vi "Test Video.vi"() -> ()   [LabVIEW 2015]
uses:
  Controls/Video Resolution Control.ctl
  Controls/Led Control.ctl
  Controls/Video Format Control.ctl
  <vilib>/Analysis/baseanly.llb/Mean (DBL).vi
  <vilib>/myRIO/Common/Instrument Driver Framework/myRIO v1.0/UART/vis/myRIO v1.0 Close UART.vi
  <vilib>/myRIO/Common/Instrument Driver Framework/Utilities/vis/FPGA Ref Manager.vi
  <vilib>/myRIO/Common/Instrument Driver Framework/myRIO v1.0/myRIO v1.0 Reset FPGA.vi
  <vilib>/myRIO/Common/Instrument Driver Framework/myRIO v1.0/IRQ/vis/myRIO v1.0 IRQ Info FGV.vi
  <vilib>/myRIO/Common/Instrument Driver Framework/myRIO v1.0/IRQ/vis/myRIO v1.0 Timer IRQ Info FGV.vi
  <vilib>/myRIO/Common/Instrument Driver Framework/myRIO v1.0/IRQ/vis/myRIO v1.0 ISR Agent.vi
  <vilib>/myRIO/Instrument Drivers/Utilities/Utilities.lvlib
  <vilib>/Analysis/NI_AALBase.lvlib
panel:
  out "Video":T1(plugin-control)
  out "period":u32
  out "mean":dbl format="%0.2f"
  in  "stop":bool
  in  "Video Res":T2
  # "LOW not working"
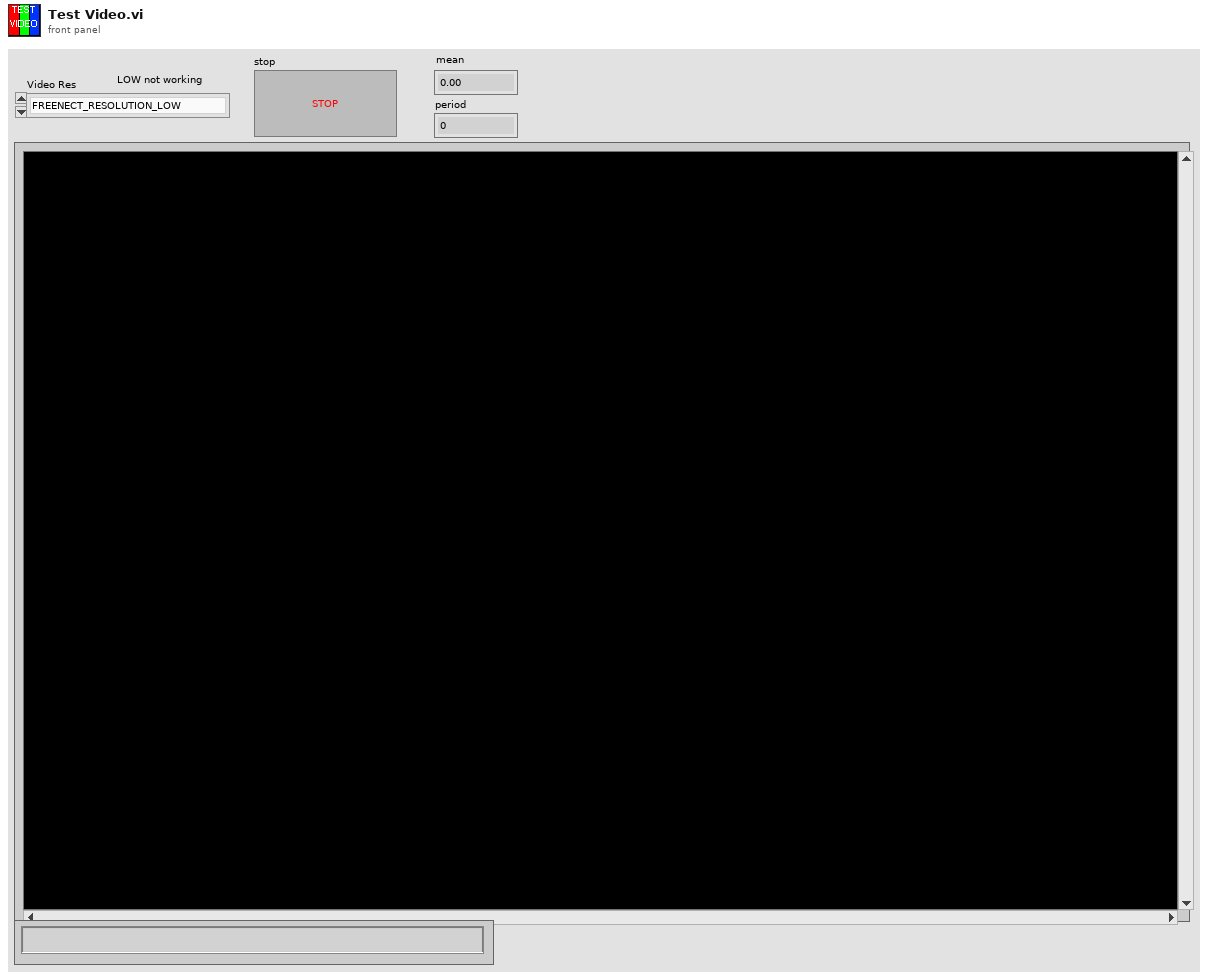
[diagram p1: front panel]
types:
  T1 = typedef "IMAQ Image.ctl" = refnum<image>
  T2 = typedef "Video Resolution Control.ctl" = enum32{"FREENECT_RESOLUTION_LOW", "FREENECT_RESOLUTION_MEDIUM", "FREENECT_RESOLUTION_HIGH"}
  T3 = enum32{"FREENECT_DEPTH_11BIT", "FREENECT_DEPTH_10BIT", "FREENECT_DEPTH_11BIT_PACKED", "FREENECT_DEPTH_10BIT_PACKED", "FREENECT_DEPTH_REGISTERED", "FREENECT_DEPTH_MM"}
  T4 = typedef "Video Format Control.ctl" = enum32{"FREENECT_VIDEO_RGB", "FREENECT_VIDEO_BAYER", "FREENECT_VIDEO_IR_8BIT", "FREENECT_VIDEO_IR_10BIT", "FREENECT_VIDEO_IR_10BIT_PACKED", "FREENECT_VIDEO_YUV_RGB", "FREENECT_VIDEO_YUV_RAW"}
  T5 = typedef "Led Control.ctl" = enum32{"LED_OFF", "LED_GREEN", "LED_RED", "LED_YELLOW", "LED_BLINK_GREEN", "LED_BLINK_GREEN2", "LED_BLINK_RED_YELLOW"}
  T6 = typedef "Image Type" = u32
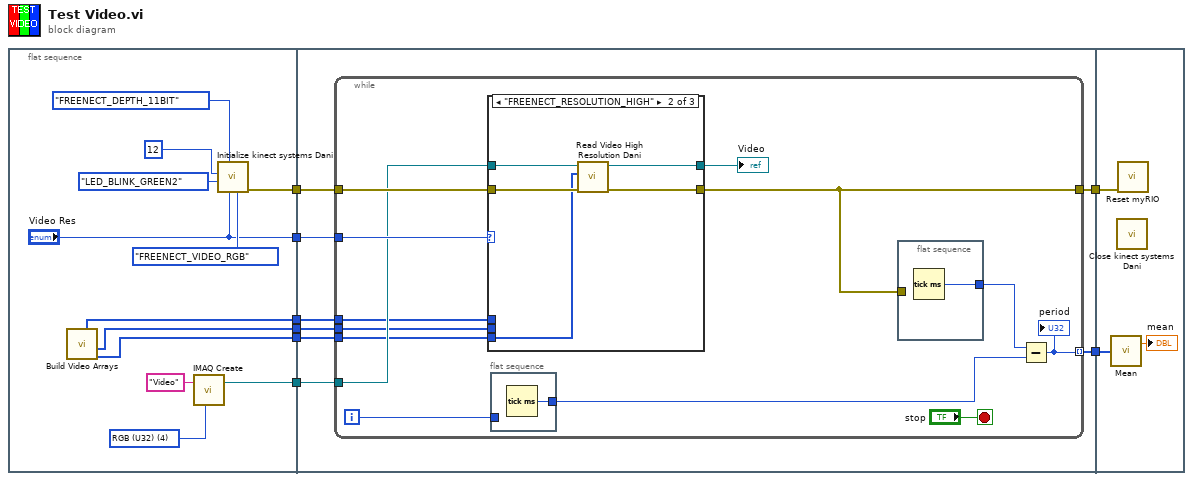
[diagram p0: block diagram]
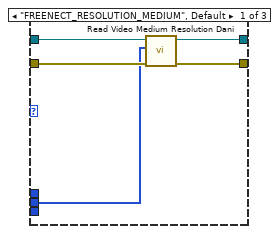
[diagram p2: hidden frame]
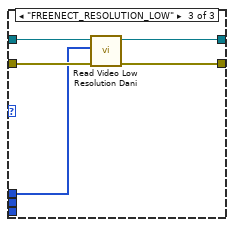
[diagram p3: hidden frame]
diagram:
  n1 = flat-sequence {
    tunnel: [w16] -> w6
    tunnel: ["Video Res"] -> w5
    tunnel: [w13] -> w4
    tunnel: [w10] -> w3
    tunnel: [w11] -> w2
    tunnel: [w9] -> w1
    tunnel: [w27] -> w8
    tunnel: [w26] -> w7
    tunnel: w6 -> [w28]
    tunnel: w5 -> [w25]
    tunnel: w4 -> [w24]
    tunnel: w3 -> [w23]
    tunnel: w2 -> [w22]
    tunnel: w1 -> [w21]
    tunnel: w8 -> [w61]
    tunnel: w7 -> [w59]
    frame #0 {
      w15 = T6 4 items=["Grayscale (U8)", "Grayscale (I16)", "Grayscale (SGL)", "Complex (CSG)", "RGB (U32)", "HSL (U32)", "RGB (U64)", "Grayscale (U16)"] ("Image Type")
      n2 = call "Build Video Arrays.vi"() -> ("Array High"=w9:u32[], "Array Medium"=w10:u32[], "Array Low"=w11:u32[])  [unwired: 9 in]
      n3 = call "IMAQ Create"("Image Name"="Video", "Image Type"=w15) -> ("New Image"=w13:T1)  [unwired: 3 in, 1 out]
      n4 = call "Initialize kinect systems Dani.vi"("Video Format"=Video_Format_Control."FREENECT_VIDEO_RGB", "Video Res"="Video Res", "Depth Format"=T3."FREENECT_DEPTH_11BIT", "Led Option"=Led_Control."LED_BLINK_GREEN2", "tilt degree"=12) -> ("error out"=w16:errorcluster)  [unwired: 6 in]
    }
    frame #1 {
      n5 = while {
        tunnel: w28 -> [w36]
        tunnel: [w37] -> w27 mode=indexing
        tunnel: [w32] -> w26
        tunnel: w25 -> [w35]
        tunnel: w24 -> [w34]
        tunnel: w23 -> [w31]
        tunnel: w22 -> [w30]
        tunnel: w21 -> [w29]
        i -> [w39]
        stop <- "stop" stop-if-true
        n6 = case shown="\"FREENECT_RESOLUTION_HIGH\"" w35 {
          tunnel: w36 -> [w46 w49 w55]
          tunnel: [w45 w50 w54] -> w32
          tunnel: [w44 w48 w53] -> w33
          tunnel: w34 -> [w43 w51 w56]
          tunnel: w31 -> [w42 _ _]
          tunnel: w30 -> [_ _ w52]
          tunnel: w29 -> [_ w47 _]
          frame "FREENECT_RESOLUTION_MEDIUM", Default {
            n7 = call "Read Video Medium Resolution Dani.vi"("error in (no error)"=w46, "video"=w42, "Image In"=w43) -> ("error out"=w45:errorcluster, "Image Out"=w44:T1)  [unwired: 7 in]
          }
          frame "FREENECT_RESOLUTION_HIGH" {
            n8 = call "Read Video High Resolution Dani.vi"("error in (no error)"=w49, "video"=w47, "Image In"=w51) -> ("error out"=w50:errorcluster, "Image Out"=w48:T1)  [unwired: 7 in]
          }
          frame "FREENECT_RESOLUTION_LOW" {
            n9 = call "Read Video Low Resolution Dani.vi"("error in (no error)"=w55, "video"=w52, "Image In"=w56) -> ("error out"=w54:errorcluster, "Image Out"=w53:T1)  [unwired: 7 in]
          }
        }
        "Video" <- w33
        n10 = flat-sequence {
          tunnel: [w57] -> w38
          tunnel: w39 -> [_]
          frame #0 {
            n11 = Tick Count (ms)() -> (millisecond timer value=w57:u32)
          }
        }
        n12 = flat-sequence {
          tunnel: [w58] -> w40
          tunnel: w32 -> [_]
          frame #0 {
            n13 = Tick Count (ms)() -> (millisecond timer value=w58:u32)
          }
        }
        n14 = Subtract(x=w40, y=w38) -> (x-y=w37:u32)
        "period" <- w37
      }
    }
    frame #2 {
      n15 = call-poly <vilib>:"Mean.vi"("X"=w61) -> ("mean"=→"mean":dbl)  [unwired: 1 out]
      n16 = call "Close kinect systems Dani.vi"() -> ()  [unwired: 11 in, 1 out]
      n17 = call <vilib>:"Reset myRIO.vi"("error in (no error)"=w59) -> ()  [unwired: 10 in, 1 out]
    }
  }
